vi "Initialize.vi"(7 "Channel Name":string="ActualValue.ch%d.AV", 8 "error in":errorcluster, 9 "Number of Channels":u32=1, 10 "Instance Name":string, 11 "Current Nominal Value in":refnum<class "Current Nominal Value.lvclass">) -> (0 "error out":errorcluster, 3 "Current Nominal Value out":refnum<class "Current Nominal Value.lvclass">)   [LabVIEW 2023, in "Current Nominal Value.lvclass"]
uses:
  Current Nominal Value.lvclass
  Current Nominal Value.lvclass/Current Nominal Value.ctl
  Parents/Nominal Value/Nominal Value.lvclass
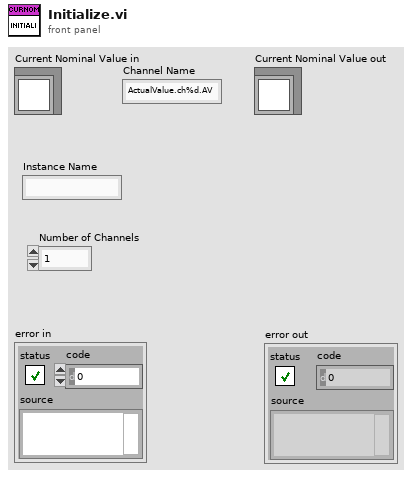
[diagram p1: front panel]
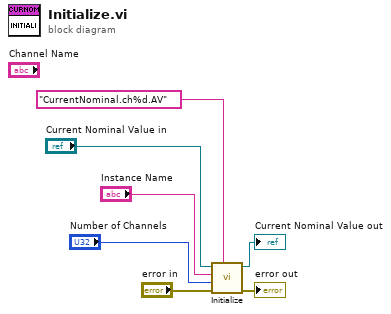
[diagram p0: block diagram]
diagram:
  n1 = call-parent "Initialize.vi"("Channel Name"="CurrentNominal.ch%d.AV" ("ChannelName"), "error in"="error in", "Number of Channels"="Number of Channels", "Instance Name"="Instance Name", "Nominal Value in"="Current Nominal Value in") -> ("error out"=→"error out":errorcluster, "Nominal Value out"=→"Current Nominal Value out":refnum<class "Current Nominal Value.lvclass">)  [unwired: 5 in]
